vi "TestAccelerometer.vi"() -> ()   [LabVIEW 2013]
panel:
  out "element":T1
  in  "stop":bool
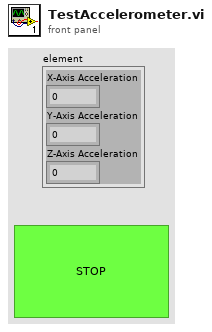
[diagram p1: front panel]
types:
  T1 = cluster{"X-Axis Acceleration":dbl, "Y-Axis Acceleration":dbl, "Z-Axis Acceleration":dbl}
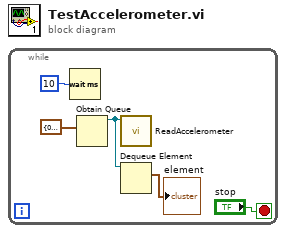
[diagram p0: block diagram]
diagram:
  n1 = while {
    stop <- "stop" stop-if-true
    n2 = Wait (ms)(milliseconds to wait=u32 10) -> ()  [unwired: 1 out]
    n3 = Obtain Queue(element data type=T1 {"X-Axis Acceleration"=0.0, "Y-Axis Acceleration"=0.0, "Z-Axis Acceleration"=0.0} ("output cluster")) -> (queue out=w2:refnum<queue>)  [unwired: 4 in, 2 out]
    n4 = call "ReadAccelerometer.vi"("Accelerometer Queue"=w2) -> ()  [unwired: 10 in, 1 out]
    n5 = Dequeue Element(queue=w2) -> (element=→"element":T1)  [unwired: 2 in, 3 out]
  }
